vi "Drive for Time.vi"(6 "Synchronization":enum16{"Start", "Wait"}(ring), 7 "Description":string, 8 "Command Info In":T1, 9 "Seconds":dbl, 10 "Right Speed":dbl, 11 "Left Speed":dbl) -> (0 "Command Info Out":T1)   [LabVIEW 2019]
doc: "This VI sets the motors to run for a given number of seconds. It optionally synchronizes with the completion of the command."
uses:
  <vilib>/Rock Robotics/WPI/Framework/Command Status Info.ctl
  <vilib>/Rock Robotics/WPI/Framework/Completion Status.ctl
  <vilib>/Rock Robotics/WPI/Framework/Completion Notifier.ctl
  Implementation/Drive Setpoints.ctl
  Implementation/Drive Operations.ctl
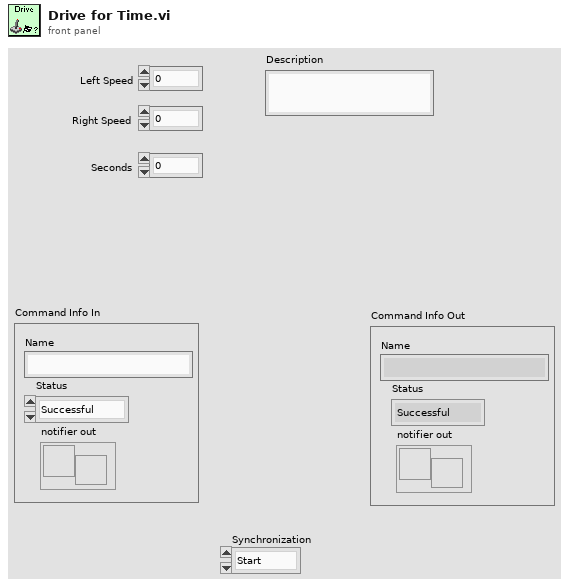
[diagram p1: front panel]
types:
  T1 = typedef "Command Status Info.ctl" = cluster{"Name":string, "Status":T2, "notifier out":T3}
  T2 = typedef "Completion Status.ctl" = enum16{"Successful", "Aborted", "Incomplete"}
  T3 = typedef "Completion Notifier.ctl" = refnum<notifier>
  T4 = typedef "Drive Setpoints.ctl" = cluster{"Operation":T5, "Left joystick x":dbl, "Left joystick y":dbl, "Duration":dbl, "Right joystick x":dbl}
  T5 = typedef "Drive Operations.ctl" = enum16{"Reserve", "Drive Immediate with Angle Control", "Read Current", "Immediate", "Drive for Time", "Drive for Distance"}
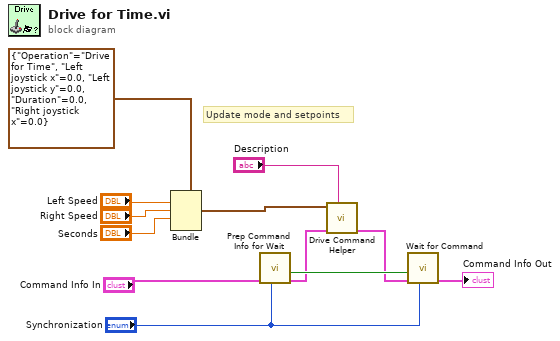
[diagram p0: block diagram]
diagram:
  # "Update mode and setpoints"
  n1 = Bundle(cluster=T4 {"Operation"=enum."Drive for Time", "Left joystick x"=0.0, "Left joystick y"=0.0, "Duration"=0.0, "Right joystick x"=0.0} ("SubSystem Data"), "Left joystick x"="Left Speed", "Left joystick y"="Right Speed", "Duration"="Seconds") -> (w4:T4)  [unwired: 2 in]
  n2 = call <vilib>:"Prep Command Info for Wait.vi"("Synchronication"="Synchronization", "Command Info"="Command Info In") -> ("Command Info"=w8:T1, "Allocated"=w9:bool)  [unwired: 8 in]
  n3 = call "Drive Command Helper.vi"("Description"="Description", "Command Info In"=w8, "SubSystem Data"=w4) -> ("Command Info Out"=w5:T1)  [unwired: 6 in, 2 out]
  n4 = call <vilib>:"Wait for Command.vi"("Synchronication"="Synchronization", "Command Info in"=w5, "Allocated"=w9) -> ("Command Info out"=→"Command Info Out":T1)  [unwired: 8 in]
